vi "Charger_Update Status Message.vi"(5 "Status Refnum":T1, 6 "error in":errorcluster, 7 "append time (T)":bool=TRUE, 8 "enable (T)":bool=TRUE, 9 "status message":string="New source.") -> (0 "error out":errorcluster)   [LabVIEW 2020]
doc: "This function writes the status message to the Error cluster source field and to the Status cluster status field.\n It includes an option to append the current time. It will not overwrite an Error cluster with an existing error."
uses:
  Charger_Status Refnum.ctl
  Drivers/Charger Test Set/Charger_Input Control.ctl
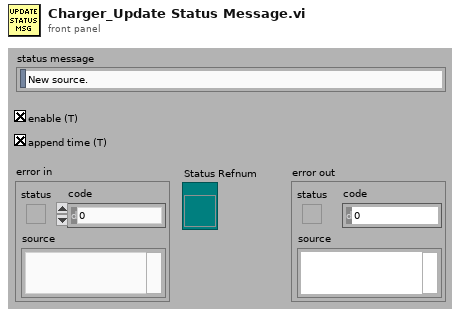
[diagram p1: front panel]
types:
  T1 = typedef "Charger_Status Refnum.ctl" = refnum<vi>
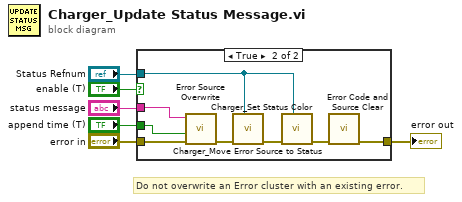
[diagram p0: block diagram]
diagram:
  # "Do not overwrite an Error cluster with an existing error."
  n1 = case shown="True" "enable (T)" {
    tunnel: "status message" -> [_ w15]
    tunnel: "append time (T)" -> [_ w13]
    tunnel: [w7 w12] -> w4
    tunnel: "error in" -> [w7 w14]
    tunnel: "Status Refnum" -> [_ w10]
    frame False {
    }
    frame True {
      n2 = call "Error Source Overwrite.vi"("error in"=w14, "append time (T)"=w13, "source"=w15) -> ("error out"=w9:errorcluster)  [unwired: 6 in]
      n3 = call "Charger_Move Error Source to Status.vi"("error in"=w9, "Status Refnum"=w10) -> ("error out"=w8:errorcluster)  [unwired: 8 in]
      n4 = call "Charger_Set Status Color.vi"("error in"=w8, "Status Refnum"=w10) -> ("error out"=w11:errorcluster)  [unwired: 8 in]
      n5 = call "Error Code and Source Clear.vi"("error in"=w11) -> ("error out"=w12:errorcluster)  [unwired: 8 in]
    }
  }
  "error out" <- w4
